vi "Archery_name.vi"() -> (0 "Enter Name Ind":string)   [LabVIEW 2014]
panel:
  in  "OK Button":bool
  in  "Enter Name":string
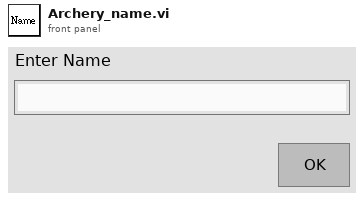
[diagram p1: front panel]
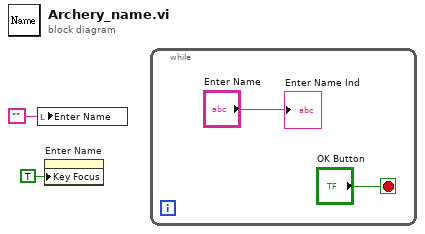
[diagram p0: block diagram]
diagram:
  n1 = local write "Enter Name"("") -> ()
  n2 = property on="Enter Name" class="Str"("Key Focus"=TRUE) -> ()  [unwired: 2 in, 2 out]
  n3 = while {
    stop <- "OK Button" stop-if-true
    "Enter Name Ind" <- "Enter Name"
  }
